vi "APU 1.0 Write Inputs.vi"(5 "Device inputs":dbl[](array[numeric]), 7 "Last Device inputs":dbl[](array[numeric]), 8 "error in (no error)":errorcluster, 9 "input reference in":T1, 10 "input in":T2, 11 "FIFO indexes.inputs":cluster{"desired speed":i32, "reset":i32}) -> (0 "error out":errorcluster, 1 "input reference out":T1, 2 "input out":T2)   [LabVIEW 2020, in "Engine Simulation Toolkit Engine.lvlib"]
uses:
  Engine Simulation Toolkit Engine.lvlib
  APU 1.0 Input Ref.ctl
  Shared/Engine Simulation Toolkit Shared.lvlib
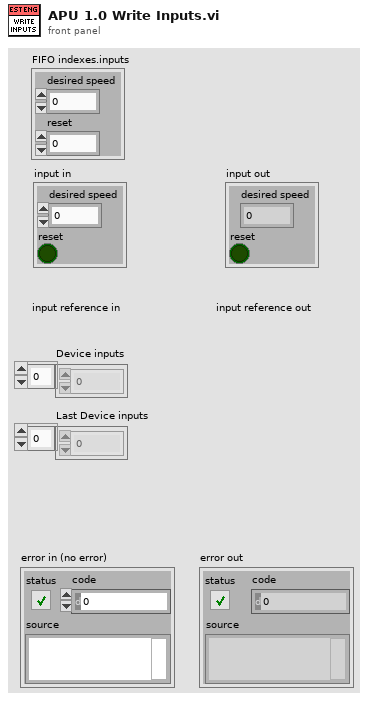
[diagram p1: front panel]
types:
  T1 = typedef "Engine Simulation Toolkit Engine.lvlib/APU 1.0 Input Ref.ctl" = refnum<k20>
  T2 = cluster{"desired speed":fxp<+/-,23,2>, "reset":bool}
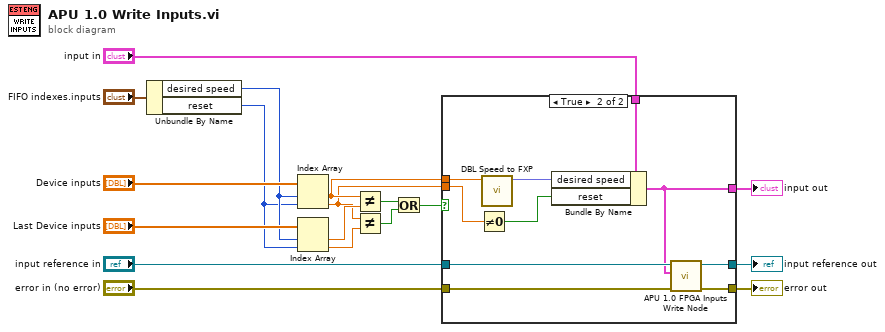
[diagram p0: block diagram]
diagram:
  n1 = Unbundle By Name("FIFO indexes.inputs") -> ("desired speed"=w10:i32, "reset"=w9:i32)
  n2 = Index Array(array="Device inputs", index #1=w10, index #2=w9) -> (element #1=w2:dbl, element #2=w1:dbl)
  n3 = Index Array(array="Last Device inputs", index #1=w10, index #2=w9) -> (element #1=w4:dbl, element #2=w3:dbl)
  n4 = Not Equal?(x=w2, y=w4) -> (x != y?=w8:bool)
  n5 = Not Equal?(x=w1, y=w3) -> (x != y?=w7:bool)
  n6 = Or(x=w8, y=w7) -> (x .or. y?=w5:bool)
  n7 = case shown="True" w5 {
    tunnel: "error in (no error)" -> [w19 w31]
    tunnel: "input reference in" -> [w20 w30]
    tunnel: [w19 w29] -> w16
    tunnel: [w20 w28] -> w15
    tunnel: "input in" -> [w21 w27]
    tunnel: [w21 w26] -> w6
    tunnel: w2 -> [_ w23]
    tunnel: w1 -> [_ w22]
    frame False {
    }
    frame True {
      n8 = Not Equal To 0?(x=w22) -> (x != 0?=w24:bool)
      n9 = call "DBL Speed to FXP.vi"("Desired speed (RPM)"=w23) -> ("FXP speed"=w25:fxp<+/-,23,2>)  [unwired: 6 in, 4 out]
      n10 = Bundle By Name(cluster=w27, "desired speed"=w25, "reset"=w24) -> (w26:T2)
      n11 = call "APU 1.0 FPGA Inputs Write Node.vi"("error in (no error)"=w31, "input in"=w26, "Refnum in"=w30) -> ("error out"=w29:errorcluster, "Refnum out"=w28:T1)  [unwired: 7 in]
    }
  }
  "error out" <- w16
  "input out" <- w6
  "input reference out" <- w15
